vi "PullData.vi"() -> ()   [LabVIEW 2009]
uses:
  <vilib>/Utility/sysdir.llb/System Directory Type.ctl
panel:
  out "DMA Mode":u8=132 format="%x"
  in  "Channel 2 Gain":T1(ring)=enum."Gain5"
  in  "Channel 2 Index":u8=1
  out "Trigger Times":u8[](array[numeric])=[0, 1, 2, 3, 4, 5, 6, 7, 8, 9, 10, 11, 12, 13, 14, 15]
  in  "Trigger Order":u8[](array[numeric])=[0, 1, 3, 4, 5, 6, 7, 8, 9, 10, 11, 6, 6, 6, 6, 6]
  in  "Channel 1 Gain":T1(ring)=enum."Gain8"
  in  "Channel 1 Index":u8
  in  "stop":bool
  out "Waveform Graph":i32[][](graph)
  in  "VISA resource name":refnum<visa-resource-name>="COM22"
  out "error out":errorcluster
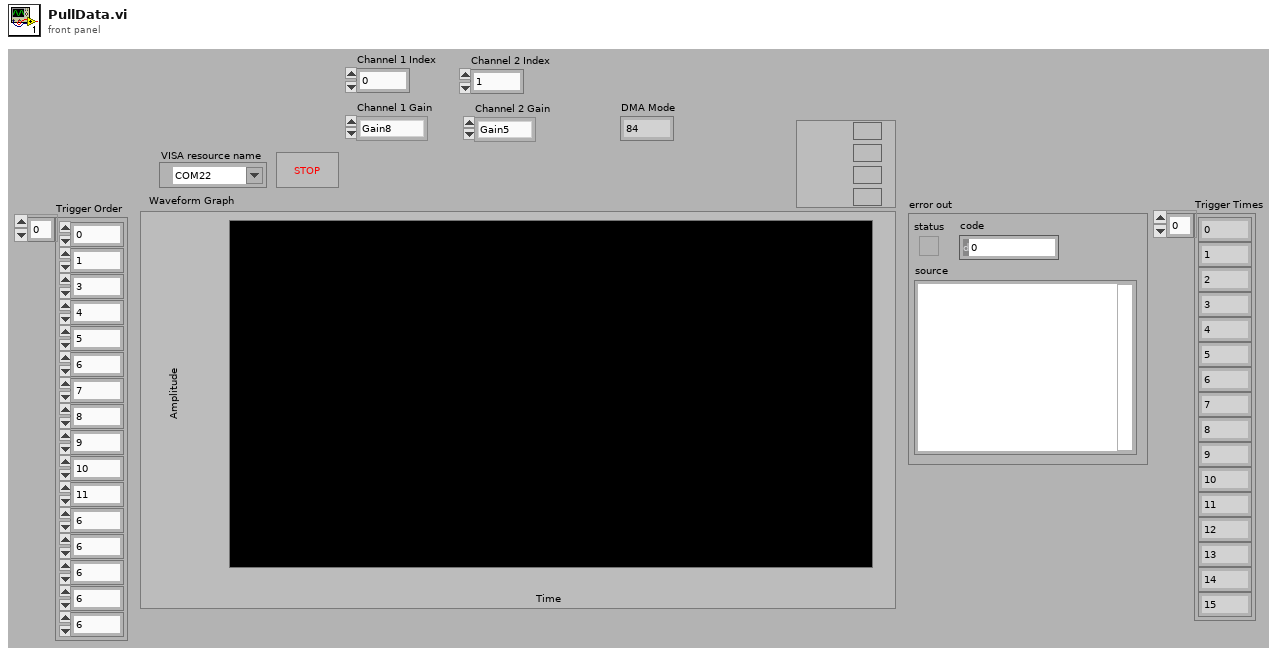
[diagram p1: front panel]
types:
  T1 = enum16{"Gain1", "Gain2", "Gain4", "Gain5", "Gain8", "Gain10", "Gain16", "Gain32", "Gain100", "Gain200", "Gain400", "Gain500", "Gain800", "Gain1000", "Gain1600", "Gain3200"}
  T2 = typedef "System Directory Type.ctl" = i32
  T3 = enum16{"open", "replace", "create", "open or create", "replace or create", "replace or create with confirmation"}
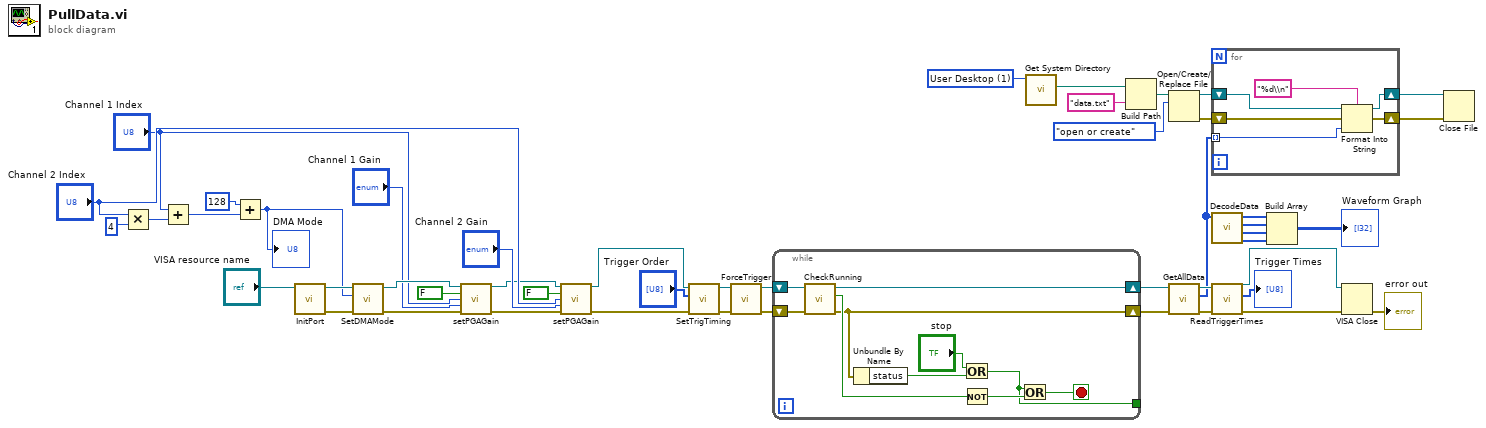
[diagram p0: block diagram]
diagram:
  w35 = T2 1 items=["User Home", "User Desktop", "User Documents", "User Application Data", "User Preferences", "User Temporary", "Public Documents", "Public Application Data", "Public Preferences", "System Core Libraries", "System Installed Libraries", "Application Files", "Boot Volume Root"] ("system directory type")
  n1 = Multiply(x="Channel 2 Index", y=u8 4) -> (x*y=w15:u8)
  n2 = Add(x="Channel 1 Index", y=w15) -> (x+y=w13:u8)
  n3 = Add(x=u8 128, y=w13) -> (x+y=w11:u8)
  "DMA Mode" <- w11
  n4 = call "InitPort.vi"("VISA resource name"="VISA resource name") -> ("error out"=w37:errorcluster, "VISA resource name out"=w36:refnum<visa-resource-name>)  [unwired: 9 in]
  n5 = call "SetDMAMode.vi"("error in (no error)"=w37, "Type"=w11, "VISA resource name"=w36) -> ("error out"=w31:errorcluster, "VISA resource name out"=w30:refnum<visa-resource-name>)  [unwired: 7 in]
  n6 = call "setPGAGain.vi"("VISA resource name"=w30, "Bank Sel"=FALSE, "Amp Index"="Channel 1 Index", "Enum"="Channel 1 Gain", "error in (no error)"=w31) -> ("VISA resource name out"=w10:refnum<visa-resource-name>, "error out"=w7:errorcluster)  [unwired: 9 in]
  n7 = call "setPGAGain.vi"("VISA resource name"=w10, "Bank Sel"=FALSE, "Amp Index"="Channel 2 Index", "Enum"="Channel 2 Gain", "error in (no error)"=w7) -> ("VISA resource name out"=w9:refnum<visa-resource-name>, "error out"=w8:errorcluster)  [unwired: 9 in]
  n8 = call "SetTrigTiming.vi"("error in (no error)"=w8, "Data"="Trigger Order", "VISA resource name"=w9) -> ("error out"=w27:errorcluster, "VISA resource name out"=w28:refnum<visa-resource-name>)  [unwired: 7 in]
  n9 = call "ForceTrigger.vi"("error in (no error)"=w27, "VISA resource name"=w28) -> ("error out"=w44:errorcluster, "VISA resource name out"=w43:refnum<visa-resource-name>)  [unwired: 8 in]
  n10 = while {
    shift-right: [w58] -> w45
    shift-left: w43 -> [w57]
    shift-right: [w53] -> w46
    shift-left: w44 -> [w56]
    tunnel: [w49] -> _
    stop <- w51 stop-if-true
    n11 = call "CheckRunning.vi"("error in (no error)"=w56, "VISA resource name"=w57) -> ("error out"=w53:errorcluster, "IsRunning"=w55:bool, "VISA resource name out"=w58:refnum<visa-resource-name>)  [unwired: 7 in]
    n12 = Unbundle By Name(w53) -> ("status"=w52:bool)
    n13 = Or(x="stop", y=w52) -> (x .or. y?=w49:bool)
    n14 = Not(x=w55) -> (.not. x?=w50:bool)
    n15 = Or(x=w49, y=w50) -> (x .or. y?=w51:bool)
  }
  n16 = call <vilib>:"Get System Directory.vi"("system directory type"=w35) -> ("system directory"=w34:path)  [unwired: 10 in]
  n17 = Build Path(base path=w34, name or relative path="data.txt") -> (appended path=w32:path)
  n18 = Open/Create/Replace File(file path (use dialog)=w32, operation (0:open)=T3."open or create") -> (refnum out=w41:refnum<file>, error out=w42:errorcluster)  [unwired: 4 in, 1 out]
  n19 = call "GetAllData.vi"("error In"=w46, "VISA resource In"=w45) -> ("error out"=w24:errorcluster, "Data Out"=w2:u16[], "VISA resource Out"=w25:refnum<visa-resource-name>)  [unwired: 7 in]
  n20 = for {
    shift-right: [w64] -> w40
    shift-left: w41 -> [w63]
    tunnel: w2 -> [w62] mode=indexing
    shift-right: [w61] -> w39
    shift-left: w42 -> [w60]
    n21 = Format Into String(format string="%d\\n", initial string=w63, error in=w60, w62) -> (resulting string=w64:refnum<file>, error out=w61:errorcluster)
  }
  n22 = call "DecodeData.vi"("Data In"=w2) -> ("Current"=w3:i16[], "Toroidal"=w4:i16[], "Poloidal"=w5:i16[], "QRatio"=w6:i32[])  [unwired: 6 in, 1 out]
  n23 = call "ReadTriggerTimes.vi"("error in (no error)"=w24, "VISA resource name"=w25) -> ("error out"=w22:errorcluster, "Data"=→"Trigger Times":u8[], "VISA resource name out"=w23:refnum<visa-resource-name>)  [unwired: 7 in]
  n24 = Build Array(w6, w5, w4, w3) -> (→"Waveform Graph":i32[][])
  n25 = VISA Close(VISA resource name=w23, error in (no error)=w22) -> (error out=→"error out":errorcluster)
  n26 = Close File(refnum=w40, error in=w39) -> ()  [unwired: 2 out]
